vi "EXO数据写入.vi"(8 "error in (no error)":errorcluster, 9 "层数":dbl, 10 "数据类型":string="N", 11 "data in":T1) -> (0 "error out":errorcluster)   [LabVIEW 2016, in "main.lvlib"]
uses:
  <vilib>/Utility/sysdir.llb/System Directory Type.ctl
  <vilib>/addons/database/Auxilliary.llb/DB Tools Transaction.ctl
  <vilib>/addons/database/Auxilliary.llb/DB Tools Isolation Level.ctl
  <vilib>/addons/database/Auxilliary.llb/DB Tools Column Info.ctl
  <vilib>/addons/database/Auxilliary.llb/DB Tools DataTypes.ctl
  <vilib>/addons/database/Auxilliary.llb/DB Tools Parameter Info.ctl
  <vilib>/addons/database/Auxilliary.llb/DB Tools Parameter Dir.ctl
  <vilib>/addons/database/Connection.llb/DB Tools Open Connec (String).vi
  <vilib>/addons/database/Connection.llb/Conn Transaction.vi
  <vilib>/addons/database/Connection.llb/Conn Execute.vi
  <vilib>/addons/database/Recordset.llb/Rec Destroy - Connection.vi
  <vilib>/addons/database/Command.llb/Cmd Set Parameter Value (C).vi
  <vilib>/addons/database/Auxilliary.llb/DB Tools Format Datetime String (Time Stamp).vi
  <vilib>/addons/database/Command.llb/Cmd Execute.vi
  <vilib>/addons/database/Recordset.llb/Rec Destroy - Command.vi
  <vilib>/addons/database/Command.llb/Cmd Delete.vi
  main.lvlib
  <vilib>/addons/database/NI_Database_API.lvlib
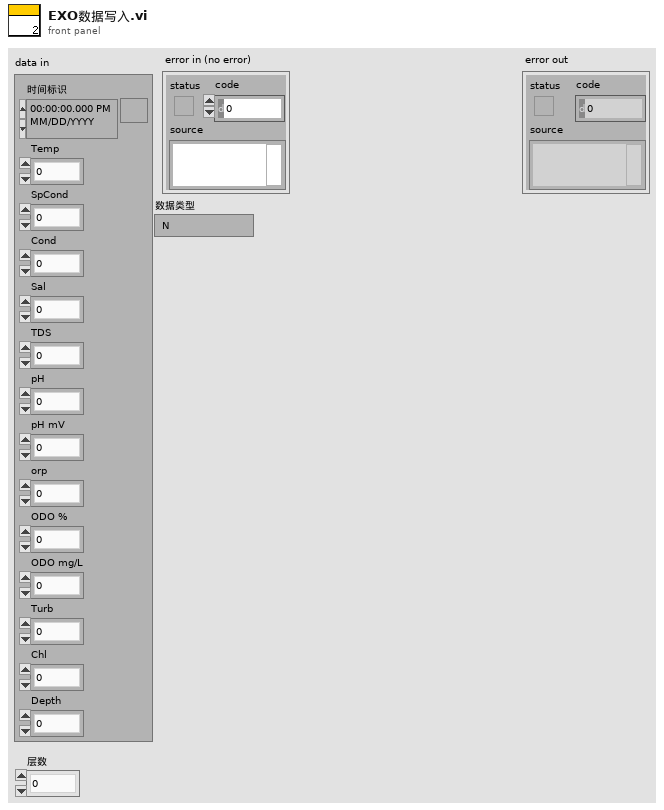
[diagram p1: front panel]
types:
  T1 = cluster{"时间标识":timestamp, "Temp":dbl, "SpCond":dbl, "Cond":dbl, "Sal":dbl, "TDS":dbl, "pH":dbl, "pH mV":dbl, "orp":dbl, "ODO %":dbl, "ODO mg/L":dbl, "Turb":dbl, "Chl":dbl, "Depth":dbl}
  T2 = typedef "NI_Database_API.lvlib/DB Tools Column Info.ctl" = cluster{"column name":string, "data type":T3, "size":i32, "allow null?":bool}
  T3 = typedef "NI_Database_API.lvlib/DB Tools DataTypes.ctl" = enum16{"String", "Long (I32)", "Single (SGL)", "Double (DBL)", "Date/Time", "Binary"}
  T4 = typedef "NI_Database_API.lvlib/DB Tools Isolation Level.ctl" = enum16{"chaos", "read uncommitted", "read committed", "repeatable read", "serializable"}
  T5 = typedef "NI_Database_API.lvlib/DB Tools Transaction.ctl" = enum16{"begin", "commit", "rollback"}
  T6 = typedef "System Directory Type.ctl" = i32
  T7 = typedef "NI_Database_API.lvlib/Conn ObjectReference.ctl" = refnum<k1>
  T8 = typedef "NI_Database_API.lvlib/DB Tools Parameter Info.ctl" = cluster{"parameter name":string, "type":T3, "direction":T9, "value":variant}
  T9 = typedef "NI_Database_API.lvlib/DB Tools Parameter Dir.ctl" = enum32{"Input", "Output", "Input/Output", "Return Value"}
  T10 = typedef "NI_Database_API.lvlib/Rec ObjectReference.ctl" = refnum<k1>
  T11 = typedef "NI_Database_API.lvlib/Cmd ObjectReference.ctl" = refnum<k1>
  T12 = typedef "NI_Database_API.lvlib/Cmd-Rec Object Reference.ctl" = refnum<k1>
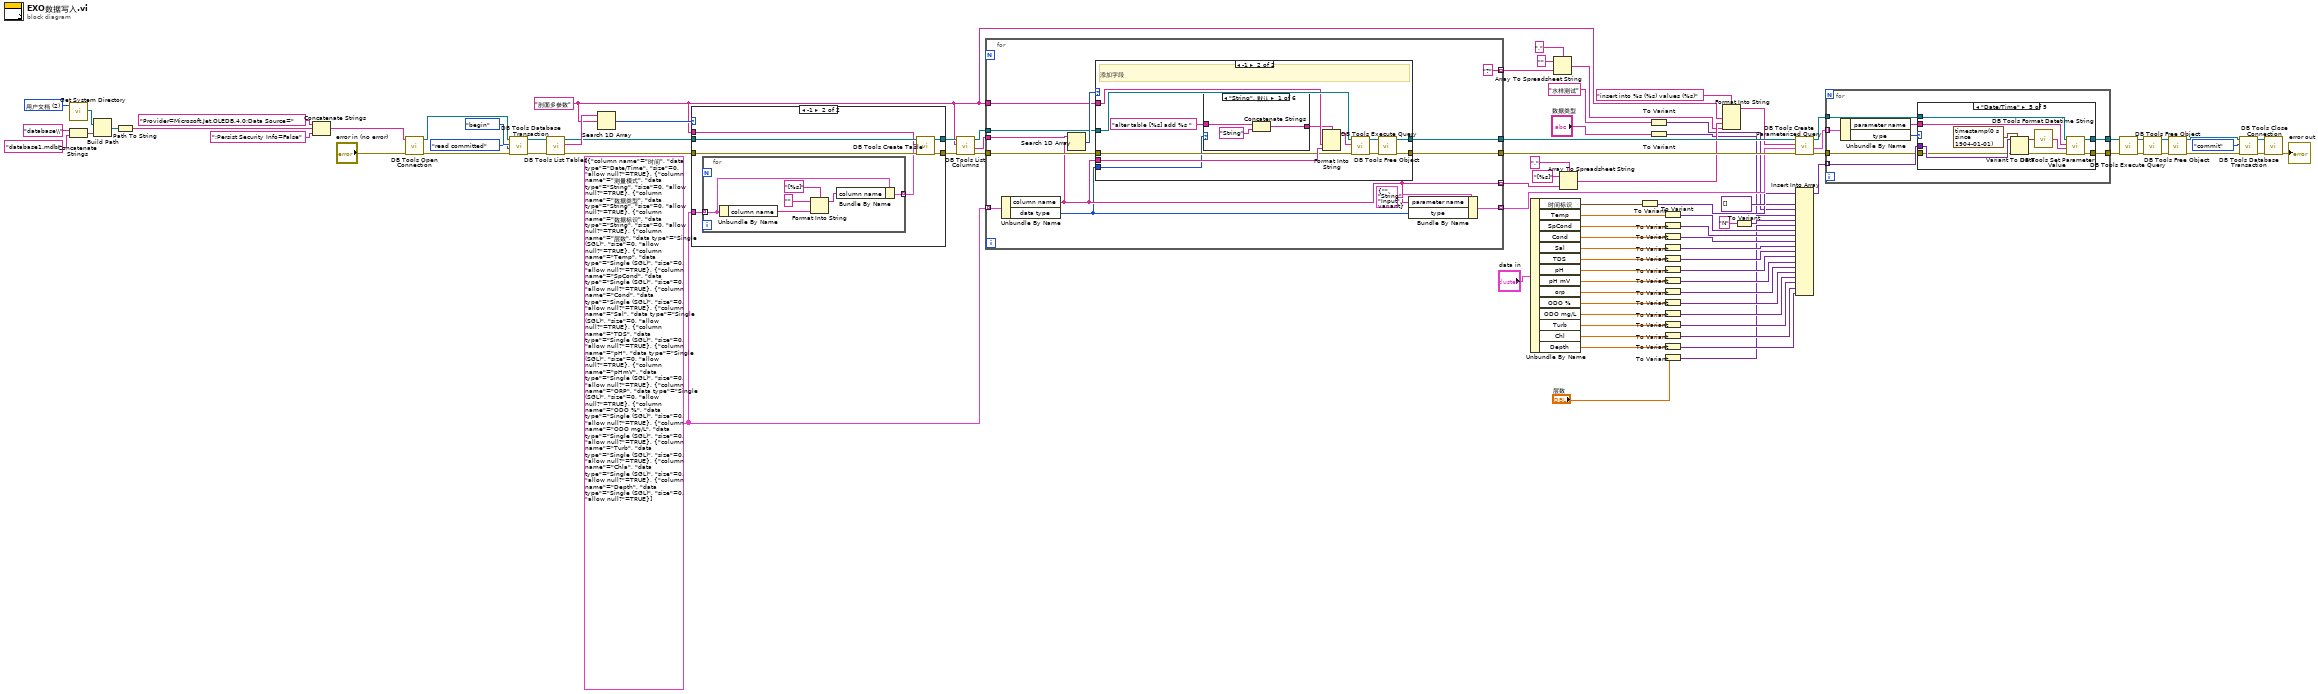
[diagram p0: block diagram]
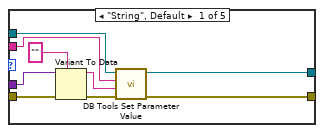
[diagram p2: hidden frame]
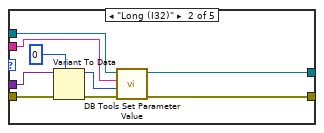
[diagram p3: hidden frame]
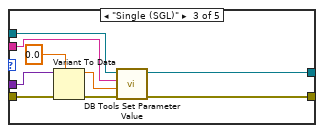
[diagram p4: hidden frame]
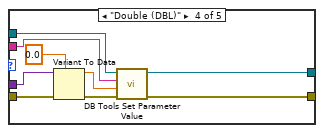
[diagram p5: hidden frame]
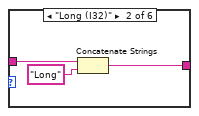
[diagram p7: hidden frame]
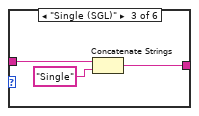
[diagram p8: hidden frame]
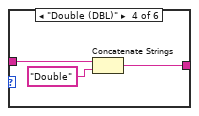
[diagram p9: hidden frame]
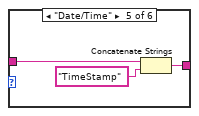
[diagram p10: hidden frame]
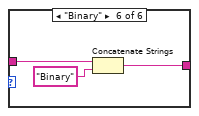
[diagram p11: hidden frame]
diagram:
  w73 = T2[] [{"column name"="时间", "data type"=enum."Date/Time", "size"=0, "allow null?"=TRUE}, {"column name"="测量模式", "data type"=enum."String", "size"=0, "allow null?"=TRUE}, {"column name"="数据类型", "data type"=enum."String", "size"=0, "allow null?"=TRUE}, {"column name"="数据标识", "data type"=enum."String", "size"=0, "allow null?"=TRUE}, {"column name"="层数", "data type"=enum."Single (SGL)", "size"=0, "allow null?"=TRUE}, {"column name"="Temp", "data type"=enum."Single (SGL)", "size"=0, "allow null?"=TRUE}, {"column name"="SpCond", "data type"=enum."Single (SGL)", "size"=0, "allow null?"=TRUE}, {"column name"="Cond", "data type"=enum."Single (SGL)", "size"=0, "allow null?"=TRUE}, {"column name"="Sal", "data type"=enum."Single (SGL)", "size"=0, "allow null?"=TRUE}, {"column name"="TDS", "data type"=enum."Single (SGL)", "size"=0, "allow null?"=TRUE}, {"column name"="pH", "data type"=enum."Single (SGL)", "size"=0, "allow null?"=TRUE}, {"column name"="pHmV", "data type"=enum."Single (SGL)", "size"=0, "allow null?"=TRUE}, {"column name"="ORP", "data type"=enum."Single (SGL)", "size"=0, "allow null?"=TRUE}, {"column name"="ODO %", "data type"=enum."Single (SGL)", "size"=0, "allow null?"=TRUE}, {"column name"="ODO mg/L", "data type"=enum."Single (SGL)", "size"=0, "allow null?"=TRUE}, {"column name"="Turb", "data type"=enum."Single (SGL)", "size"=0, "allow null?"=TRUE}, {"column name"="Chla", "data type"=enum."Single (SGL)", "size"=0, "allow null?"=TRUE}, {"column name"="Depth", "data type"=enum."Single (SGL)", "size"=0, "allow null?"=TRUE}] ("column information")
  w66 = "剖面多参数"
  w95 = T6 2 items=["用户目录"=0, "用户桌面"=1, "用户文档"=2, "用户应用程序数据"=3, "用户设置"=4, "用户临时目录"=5, "公共文档"=6, "公共应用程序数据"=7, "公共设置"=8, "公共缓存"=13, "系统核心库"=9, "系统安装库"=10, "应用程序文件"=11, "启动盘根目录"=12] ("system directory type")
  n1 = call <vilib>:"Get System Directory.vi"("system directory type"=w95) -> ("system directory"=w93:path)  [unwired: 10 in]
  n2 = Concatenate Strings("database\\" ("condition"), "database1.mdb" ("database")) -> (w87:string)
  n3 = Build Path(base path=w93, name or relative path=w87) -> (appended path=w92:path)
  n4 = Path To String(path=w92) -> (string=w91:string)
  n5 = Concatenate Strings("Provider=Microsoft.Jet.OLEDB.4.0;Data Source=" ("condition"), w91, ";Persist Security Info=False" ("condition")) -> (w89:string)
  n6 = call-poly <vilib>:"DB Tools Open Connection.vi"("error in (no error)"="error in (no error)", "connection information"=w89) -> ("error out"=w36:errorcluster, "connection reference"=w38:T7)  [unwired: 6 in]
  n7 = call-poly <vilib>:"DB Tools Database Transaction.vi"("error in (no error)"=w36, "isolation level (chaos)"=DB_Tools_Isolation_Level."read committed", "operation (begin)"=DB_Tools_Transaction."begin", "connection reference"=w38) -> ("error out"=w35:errorcluster, "connection reference out"=w37:T7)  [unwired: 2 in]
  n8 = call <vilib>:"DB Tools List Tables.vi"("error in (no error)"=w35, "connection reference"=w37) -> ("error out"=w77:errorcluster, "tables"=w80:string[], "connection reference out"=w78:T7)  [unwired: 3 in]
  n9 = Search 1D Array(1D array=w80, element=w66) -> (index of element=w79:i32)  [unwired: 1 in]
  n10 = case shown="-1" w79 {
    tunnel: w78 -> [w97 w104]
    tunnel: w77 -> [w96 w103]
    tunnel: w66 -> [_ w102]
    tunnel: w73 -> [_ w99]
    tunnel: [w97 w101] -> w72
    tunnel: [w96 w100] -> w71
    frame 0, Default {
    }
    frame -1 {
      n11 = for {
        tunnel: w99 -> [w107] mode=indexing
        tunnel: [w105] -> w98 mode=indexing
        n12 = Unbundle By Name(w107) -> ("column name"=w110:string)
        n13 = Format Into String(format string="[%s]" ("格式字符串"), initial string="" ("初始字符串"), w110) -> (resulting string=w106:string)  [unwired: 1 in, 1 out]
        n14 = Bundle By Name(cluster=w107, "column name"=w106) -> (w105:T2)
      }
      n15 = call <vilib>:"DB Tools Create Table.vi"("error in (no error)"=w103, "column information"=w98, "table"=w102, "connection reference"=w104) -> ("error out"=w100:errorcluster, "connection reference out"=w101:T7)  [unwired: 4 in]
    }
  }
  n16 = call <vilib>:"DB Tools List Columns.vi"("error in (no error)"=w71, "table"=w66, "connection reference"=w72) -> ("error out"=w74:errorcluster, "columns"=w75:string[], "connection reference out"=w76:T7)  [unwired: 1 in, 1 out]
  n17 = for {
    tunnel: w76 -> [w121]
    tunnel: w75 -> [w123]
    tunnel: w74 -> [w120]
    tunnel: [w119] -> w70
    tunnel: [w118] -> w69
    tunnel: w66 -> [w117]
    tunnel: w73 -> [w116] mode=indexing
    tunnel: [w114] -> w68 mode=indexing
    tunnel: [w113] -> w61 mode=indexing
    tunnel: ["?"] -> w59 mode=indexing
    n18 = Unbundle By Name(w116) -> ("column name"=w113:string, "data type"=w111:T3)
    n19 = Search 1D Array(1D array=w123, element=w113) -> (index of element=w122:i32)  [unwired: 1 in]
    n20 = case shown="-1" w122 {
      tunnel: [w125 w134] -> w118
      tunnel: [w124 w133] -> w119
      tunnel: w121 -> [w125 w132]
      tunnel: w113 -> [_ w131]
      tunnel: w120 -> [w124 w130]
      tunnel: w117 -> [_ w129]
      tunnel: w111 -> [_ w127]
      frame 0, Default {
      }
      frame -1 {
        # "添加字段"
        n21 = case shown="\"String\", 默认" w127 {
          tunnel: "alter table [%s] add %s " -> [w140 w143 w146 w149 w152 w155]
          tunnel: [w139 w142 w145 w148 w151 w154] -> w126
          frame "String", Default {
            n22 = Concatenate Strings(w140, "String" ("字符串")) -> (w139:string)
          }
          frame "Long (I32)" {
            n23 = Concatenate Strings(w143, "Long" ("字符串")) -> (w142:string)
          }
          frame "Single (SGL)" {
            n24 = Concatenate Strings(w146, "Single" ("字符串")) -> (w145:string)
          }
          frame "Double (DBL)" {
            n25 = Concatenate Strings(w149, "Double" ("字符串")) -> (w148:string)
          }
          frame "Date/Time" {
            n26 = Concatenate Strings(w152, "TimeStamp" ("字符串")) -> (w151:string)
          }
          frame "Binary" {
            n27 = Concatenate Strings(w155, "Binary" ("字符串")) -> (w154:string)
          }
        }
        n28 = Format Into String(format string=w126, w129, w131) -> (resulting string=w135:string)  [unwired: 2 in, 1 out]
        n29 = call-poly <vilib>:"DB Tools Execute Query.vi"("error in (no error)"=w130, "SQL query"=w135, "connection reference"=w132) -> ("error out"=w136:errorcluster, "recordset reference"=w137:T10)  [unwired: 5 in]
        n30 = call-poly <vilib>:"DB Tools Free Object.vi"("error in (no error)"=w136, "recordset reference"=w137) -> ("error out"=w133:errorcluster, "connection reference"=w134:T7)  [unwired: 8 in]
      }
    }
    n31 = Bundle By Name(cluster=T8 {"parameter name"="", "type"=enum."String", "direction"=enum."Input", "value"=variant} ("parameter information"), "parameter name"=w113, "type"=w111) -> (w114:T8)
  }
  n32 = Unbundle By Name("data in") -> ("时间标识"=w53:timestamp, "Temp"=w52:dbl, "SpCond"=w33:dbl, "Cond"=w32:dbl, "Sal"=w31:dbl, "TDS"=w30:dbl, "pH"=w29:dbl, "pH mV"=w28:dbl, "orp"=w27:dbl, "ODO %"=w26:dbl, "ODO mg/L"=w25:dbl, "Turb"=w24:dbl, "Chl"=w23:dbl, "Depth"=w22:dbl)
  n33 = Array To Spreadsheet String(delimiter (Tab)="," ("分隔符(Tab)"), array=w59, 3:"" ("格式字符串")) -> (spreadsheet string=w58:string)
  n34 = Array To Spreadsheet String(delimiter (Tab)="," ("分隔符(Tab)"), array=w61, 3:"[%s]" ("格式字符串")) -> (spreadsheet string=w60:string)
  n35 = To Variant(anything=w53) -> (Variant=w9:variant)
  n36 = To Variant(anything="水样测试") -> (Variant=w8:variant)
  n37 = To Variant(anything="数据类型") -> (Variant=w3:variant)
  n38 = To Variant(anything=w52) -> (Variant=w50:variant)
  n39 = To Variant(anything=w33) -> (Variant=w21:variant)
  n40 = To Variant(anything=w32) -> (Variant=w20:variant)
  n41 = To Variant(anything=w31) -> (Variant=w19:variant)
  n42 = To Variant(anything=w30) -> (Variant=w18:variant)
  n43 = To Variant(anything=w29) -> (Variant=w17:variant)
  n44 = To Variant(anything=w28) -> (Variant=w16:variant)
  n45 = To Variant(anything=w27) -> (Variant=w15:variant)
  n46 = To Variant(anything=w26) -> (Variant=w14:variant)
  n47 = To Variant(anything=w25) -> (Variant=w13:variant)
  n48 = To Variant(anything=w24) -> (Variant=w12:variant)
  n49 = To Variant(anything=w23) -> (Variant=w11:variant)
  n50 = To Variant(anything=w22) -> (Variant=w10:variant)
  n51 = To Variant(anything="层数") -> (Variant=w2:variant)
  n52 = Format Into String(format string="insert into %s (%s) values (%s)" ("格式字符串"), w66, w60, w58) -> (resulting string=w57:string)  [unwired: 2 in, 1 out]
  n53 = To Variant(anything="N") -> (Variant=w5:variant)
  n54 = call <vilib>:"DB Tools Create Parameterized Query.vi"("error in (no error)"=w70, "parameters"=w68, "SQL query"=w57, "connection reference"=w69) -> ("error out"=w55:errorcluster, "parameters out"=w54:T8[], "command reference"=w56:T11)  [unwired: 3 in]
  n55 = Insert Into Array(array=variant[] [], new element #1=w9, new element #2=w8, new element #3=w3, new element #4=w5, new element #5=w2, new element #6=w50, new element #7=w21, new element #8=w20, new element #9=w19, new element #10=w18, new element #11=w17, new element #12=w16, new element #13=w15, new element #14=w14, new element #15=w13, new element #16=w12, new element #17=w11, new element #18=w10) -> (w49:variant[])  [unwired: 1 in]
  n56 = for {
    tunnel: w56 -> [w160]
    tunnel: w55 -> [w158]
    tunnel: w54 -> [w163] mode=indexing
    tunnel: w49 -> [w161] mode=indexing
    tunnel: [w157] -> w48
    tunnel: [w156] -> w47
    n57 = Unbundle By Name(w163) -> ("parameter name"=w159:string, "type"=w162:T3)
    n58 = case shown="\"Date/Time\"" w162 {
      tunnel: w161 -> [w167 w175 w182 w192 w209]
      tunnel: w160 -> [w170 w179 w186 w196 w207]
      tunnel: w159 -> [w169 w178 w185 w191 w206]
      tunnel: w158 -> [w164 w173 w183 w193 w204]
      tunnel: [w166 w177 w187 w195 w203] -> w157
      tunnel: [w165 w176 w184 w194 w202] -> w156
      frame "String", Default {
        n59 = Variant To Data(error in=w164, type="", Variant=w167) -> (data=w168:string, error out=w172:errorcluster)
        n60 = call-poly <vilib>:"DB Tools Set Parameter Value.vi"("error in (no error)"=w172, "value"=w168, "parameter index"=w169, "command reference"=w170) -> ("error out"=w165:errorcluster, "command reference out"=w166:T11)  [unwired: 4 in]
      }
      frame "Long (I32)" {
        n61 = Variant To Data(error in=w173, type=0, Variant=w175) -> (data=w180:i32, error out=w181:errorcluster)
        n62 = call-poly <vilib>:"DB Tools Set Parameter Value.vi"("error in (no error)"=w181, "value"=w180, "parameter index"=w178, "command reference"=w179) -> ("error out"=w176:errorcluster, "command reference out"=w177:T11)  [unwired: 4 in]
      }
      frame "Single (SGL)" {
        n63 = Variant To Data(error in=w183, type=sgl 0.0, Variant=w182) -> (data=w189:sgl, error out=w190:errorcluster)
        n64 = call-poly <vilib>:"DB Tools Set Parameter Value.vi"("error in (no error)"=w190, "value"=w189, "parameter index"=w185, "command reference"=w186) -> ("error out"=w184:errorcluster, "command reference out"=w187:T11)  [unwired: 4 in]
      }
      frame "Double (DBL)" {
        n65 = Variant To Data(error in=w193, type=0.0, Variant=w192) -> (data=w198:dbl, error out=w199:errorcluster)
        n66 = call-poly <vilib>:"DB Tools Set Parameter Value.vi"("error in (no error)"=w199, "value"=w198, "parameter index"=w191, "command reference"=w196) -> ("error out"=w194:errorcluster, "command reference out"=w195:T11)  [unwired: 4 in]
      }
      frame "Date/Time" {
        n67 = Variant To Data(error in=w204, type=timestamp(0 s since 1904-01-01) ("时间标识"), Variant=w209) -> (data=w201:timestamp, error out=w205:errorcluster)
        n68 = call-poly <vilib>:"DB Tools Format Datetime String.vi"("time stamp"=w201) -> ("date/time string"=w200:string)
        n69 = call-poly <vilib>:"DB Tools Set Parameter Value.vi"("error in (no error)"=w205, "value"=w200, "parameter index"=w206, "command reference"=w207) -> ("error out"=w202:errorcluster, "command reference out"=w203:T11)  [unwired: 4 in]
      }
    }
  }
  n70 = call-poly <vilib>:"DB Tools Execute Query.vi"("error in (no error)"=w47, "command reference"=w48) -> ("error out"=w45:errorcluster, "command-recordset reference"=w46:T12)  [unwired: 6 in]
  n71 = call-poly <vilib>:"DB Tools Free Object.vi"("error in (no error)"=w45, "command-recordset reference"=w46) -> ("error out"=w43:errorcluster, "command reference"=w44:T11)  [unwired: 8 in]
  n72 = call-poly <vilib>:"DB Tools Free Object.vi"("error in (no error)"=w43, "command reference"=w44) -> ("error out"=w39:errorcluster, "connection reference"=w40:T7)  [unwired: 8 in]
  n73 = call-poly <vilib>:"DB Tools Database Transaction.vi"("error in (no error)"=w39, "operation (begin)"=DB_Tools_Transaction."commit", "connection reference"=w40) -> ("error out"=w41:errorcluster, "connection reference out"=w42:T7)  [unwired: 3 in]
  n74 = call <vilib>:"DB Tools Close Connection.vi"("error in (no error)"=w41, "connection reference"=w42) -> ("error out"=→"error out":errorcluster)  [unwired: 5 in]
